vi "Read Category Name.vi"(8 "error in (no error)":errorcluster, 11 "Config Plugin in":refnum<class "Config Plugin.lvclass">) -> (0 "error out":errorcluster, 2 "Category Name":string, 3 "Config Plugin out":refnum<class "Config Plugin.lvclass">)   [LabVIEW 2016, in "Config Plugin.lvlib" / "Config Plugin.lvclass"]
uses:
  <userlib>/Common Components/Config Plugin/Config Plugin.lvclass
  <userlib>/Common Components/Config Plugin/Config Plugin.lvclass/Config Plugin.ctl
  <userlib>/_OpenG.lib/file/file.llb/Strip Path Extension - String__ogtk.vi
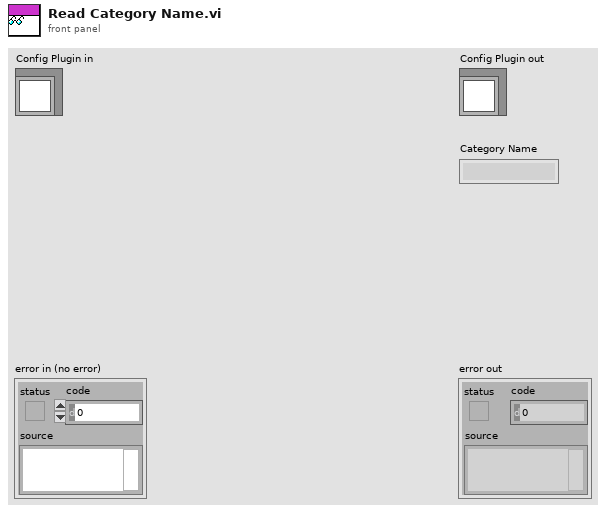
[diagram p1: front panel]
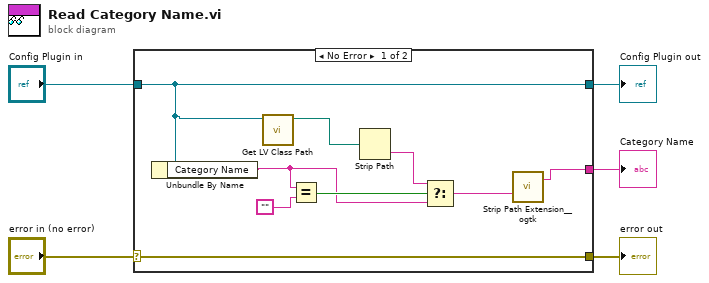
[diagram p0: block diagram]
diagram:
  n1 = case shown="No Error" "error in (no error)" {
    selector: "error in (no error)" -> [w14 w15]
    tunnel: [w14 w15] -> w4
    tunnel: [w8 w16] -> w2
    tunnel: "Config Plugin in" -> [w8 w16]
    tunnel: [w6 _] -> w1
    frame No Error {
      n2 = Unbundle By Name(w8) -> ("Category Name"=w7:string)
      n3 = call <vilib>:"Get LV Class Path.vi"("object"=w8) -> ("class path"=w10:path)  [unwired: 9 in, 1 out]
      n4 = Equal?(x=w7, y="") -> (x = y?=w12:bool)
      n5 = Strip Path(path=w10) -> (name=w11:string)  [unwired: 1 out]
      n6 = Select(t=w11, s=w12, f=w7) -> (s? t:f=w9:string)
      n7 = call-poly <userlib>:"Strip Path Extension__ogtk.vi"("path"=w9) -> ("root"=w6:string)  [unwired: 1 out]
    }
    frame Error {
    }
  }
  "error out" <- w4
  "Config Plugin out" <- w2
  "Category Name" <- w1
